vi "Init all motors.vi"() -> (3 "AISAS Motors":refnum<class "AISAS motor.lvclass">[](array[class]))   [LabVIEW 2014, in "AISAS motor.lvclass"]
uses:
  AISAS motor.lvclass
  Controls/motor.ctl
  AISAS motor.lvclass/AISAS motor.ctl
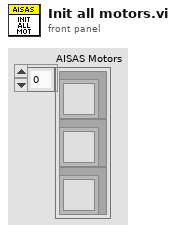
[diagram p1: front panel]
types:
  T1 = typedef "motor.ctl" = enum32{"Rotation", "Diffuser ", "Focus"}
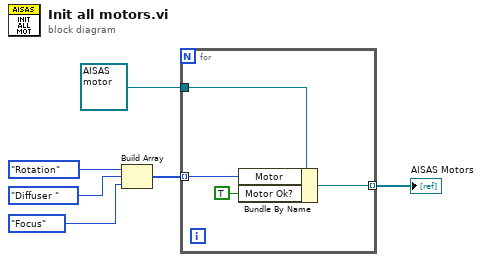
[diagram p0: block diagram]
diagram:
  n1 = Build Array(motor."Rotation" ("Motor"), motor."Diffuser " ("Motor"), motor."Focus" ("Motor")) -> (w3:T1[])
  n2 = for {
    tunnel: w3 -> [w8] mode=indexing
    tunnel: refnum<class "AISAS motor.lvclass"> refnum ("AISAS control.lvclass") -> [w10]
    tunnel: [w9] -> w1 mode=indexing
    n3 = Bundle By Name(cluster=w10, "Motor"=w8, "Motor Ok?"=TRUE) -> (w9:refnum<class "AISAS motor.lvclass">)
  }
  "AISAS Motors" <- w1
